vi "Divide.vi"(8 "Error In":errorcluster, 10 "y":dbl, 11 "x":dbl) -> (0 "Error Out":errorcluster, 3 "z":dbl)   [LabVIEW 2025]
doc: "Use the LabVIEW Unit Test Framework Toolkit to check this VI for functional correctness. One test file for this VI, Divide.lvtest, is configured to contain an error. Another test file for this VI, Divide by Zero.lvtest is configured to pass, even when this VI reports an error."
panel:
  # "Overview: Use the LabVIEW Unit Test Framework Toolkit to check this VI for functional correctness.\nRequirements: LabVIEW Full Development System, Unit Test Framework Toolkit\nInstructions:\n1.  Execute the Divide.lvtest file for this VI.\n     a)  In the Project Explorer window, expand the Unit Test Files folder, right-click Divide.lvtest, and select Run from the shortcut menu.\n     b)  View the test results in the Unit Test Framework Results window, which shows that the test contains an error.\n     c)   In the Unit Test Framework Results, click the Test Errors tab, expand all the items in the Error Details pane, and click Divide.lvtest to\n           display the error description. You can find that this test reports an error because LabVIEW cannot find the output terminal of z in the VI.\n     d)  Click OK to close the window.\n     e) \t In the Project Explorer window, double-click Divide.lvtest to open the Test Properties dialog box.\n      f) \tOn the Test Cases page, click the Update button to update the inputs and output of this VI.\n     g)\t Click OK to close the dialog box.\n     h)\t In the Project Explorer window, expand the Unit Test Files folder, right-click Divide.lvtest, and select Run from the shortcut menu.\n      i)\t View the test results in the Unit Test Framework Results window, which shows that the test passes.\n2.  Execute the Divide by Zero.lvtest  file for this VI.\n     a)  In the Project Explorer window, right-click Divide by zero.lvtest, and select Run from the shortcut menu.\n     b)  View the test results in the Unit Test Framework Results window, which shows that the test passes.\n     c)  Return to this VI. You will find this VI reports an error because x is divided by zero. However, this test still passes because the value of the\n          output in this VI matches the expected value in the Divide by Zero.lvtest test file."
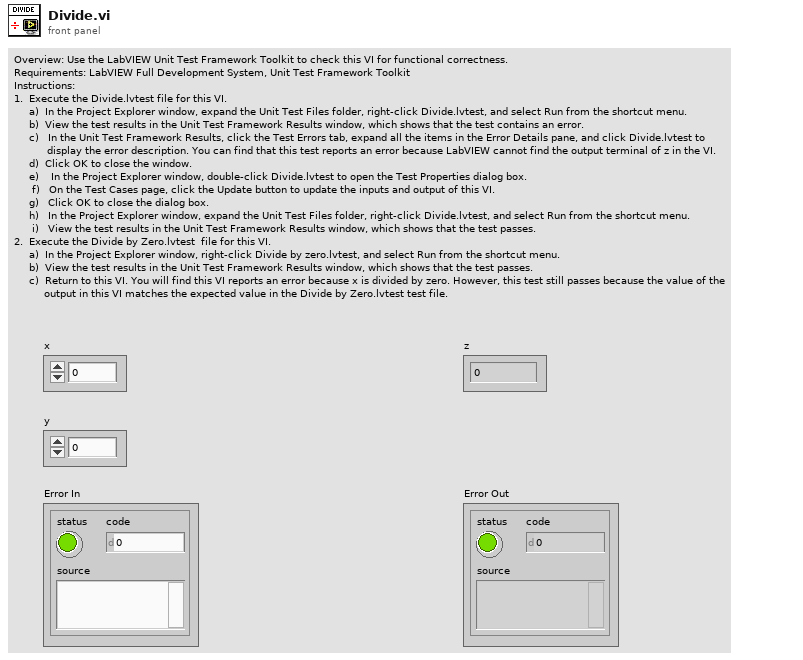
[diagram p1: front panel]
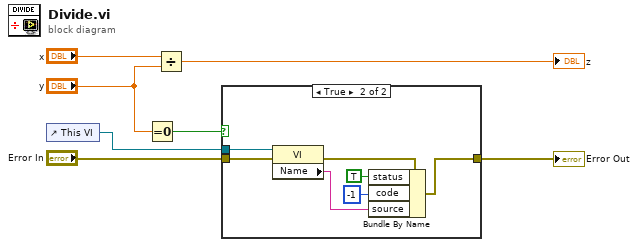
[diagram p0: block diagram]
diagram:
  n1 = control-ref of="This VI"() -> (w1:refnum<vi>)
  n2 = Equal To 0?(x="y") -> (x = 0?=w4:bool)
  n3 = Divide(x="x", y="y") -> (x/y=→"z":dbl)
  n4 = case shown="True" w4 {
    tunnel: "Error In" -> [w8 w11]
    tunnel: [w8 w13] -> w2
    tunnel: w1 -> [_ w9]
    frame False {
    }
    frame True {
      n5 = property class="VI"(reference=w9, error in=w11) -> (error out=w10:errorcluster, "Name"=w14:string)  [unwired: 1 out]
      n6 = Bundle By Name(cluster=w10, "status"=TRUE, "code"=-1, "source"=w14) -> (w13:errorcluster)
    }
  }
  "Error Out" <- w2
